vi "Configure Zone.vi"(0 "VISA resource name":refnum<visa-resource-name>, 1 "Manual\nOutput (0.000)":dbl[](array[numeric]) min=-100.0 max=100.0 step=0.001 format="%.3f", 2 "Heater\nRange (0: Off)":i8[](array[ring]) items=["Off", "Low (0.5W)", "Med (5W)", "High (50W)"], 5 "Loop (0: 1)":u16(ring) items=["1", "2"], 9 "Top \nValue (0.0000)":dbl[](array[numeric]) min=-273.0 max=1500.0 step=0.0001 format="%.4f", 11 "error in (no error)":errorcluster, 12 "Gain (0.0)":dbl[](array[numeric]) min=0.0 max=1000.0 step=0.1 format="%.1f", 13 "Reset (0.0)":dbl[](array[numeric]) min=0.0 max=1000.0 step=0.1 format="%.1f", 14 "Rate (0)":dbl[](array[numeric]) min=0.0 max=200.0 step=1.0) -> (4 "VISA resource name out":refnum<visa-resource-name>, 6 "Zone":i32[](array[numeric]) min=1 max=10 step=1, 15 "error out":errorcluster)   [LabVIEW 2013, in "Lake Shore Cryotronics 331.lvlib"]
doc: "This VI Configures the parameters of a control loop's zone table. The zone values are configured into arrays to allow all ten zones to be sent each time the vi is executed."
uses:
  Lake Shore Cryotronics 331.lvlib
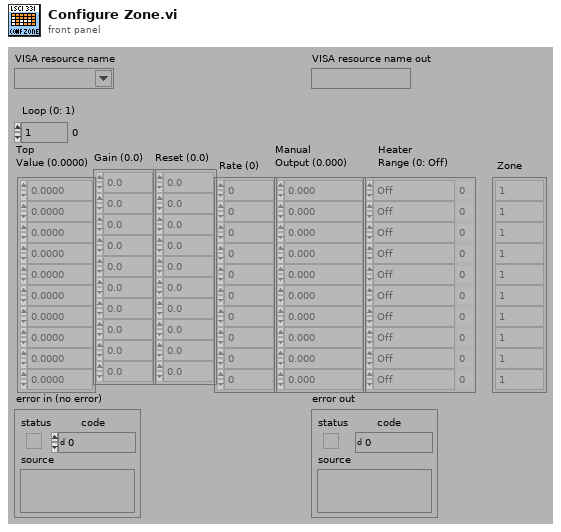
[diagram p1: front panel]
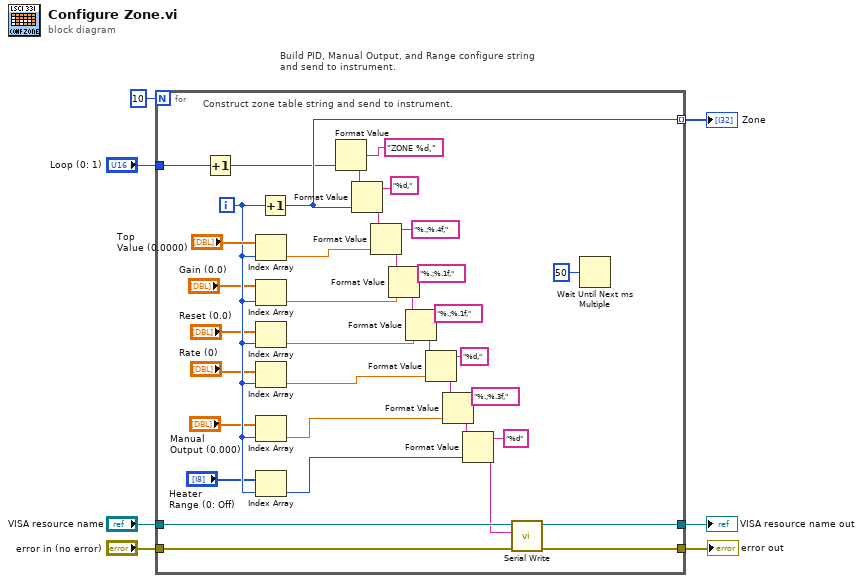
[diagram p0: block diagram]
diagram:
  # "Build PID, Manual Output, and Range configure string\nand send to instrument."
  n1 = for {
    N: 10 -> [_]
    tunnel: [w28] -> w6 mode=indexing
    tunnel: "Loop (0: 1)" -> [w25]
    tunnel: "error in (no error)" -> [w13]
    tunnel: [w12] -> w4
    tunnel: [w11] -> w3
    tunnel: "VISA resource name" -> [w9]
    i -> [w22]
    # "Construct zone table string and send to instrument."
    n2 = Increment(x=w25) -> (x+1=w10:u16)
    n3 = Index Array(array="Top \nValue (0.0000)", index=w22) -> (element=w33:dbl)
    n4 = Index Array(array="Gain (0.0)", index=w22) -> (element=w32:dbl)
    n5 = Index Array(array="Reset (0.0)", index=w22) -> (element=w31:dbl)
    n6 = Index Array(array="Rate (0)", index=w22) -> (element=w30:dbl)
    n7 = Index Array(array="Manual\nOutput (0.000)", index=w22) -> (element=w29:dbl)
    n8 = Index Array(array="Heater\nRange (0: Off)", index=w22) -> (element=w18:i8)
    n9 = Increment(x=w22) -> (x+1=w28:i32)
    n10 = Format Value(format string="ZONE %d,", value (0)=w10) -> (output string=w24:string)  [unwired: 1 in]
    n11 = Format Value(string ("")=w24, format string="%d,", value (0)=w28) -> (output string=w35:string)
    n12 = Format Value(string ("")=w35, format string="%.;%.4f,", value (0)=w33) -> (output string=w41:string)
    n13 = Format Value(string ("")=w41, format string="%.;%.1f,", value (0)=w32) -> (output string=w42:string)
    n14 = Format Value(string ("")=w42, format string="%.;%.1f,", value (0)=w31) -> (output string=w43:string)
    n15 = Format Value(string ("")=w43, format string="%d,", value (0)=w30) -> (output string=w44:string)
    n16 = Format Value(string ("")=w44, format string="%.;%.3f,", value (0)=w29) -> (output string=w19:string)
    n17 = Format Value(string ("")=w19, format string="%d", value (0)=w18) -> (output string=w8:string)
    n18 = call "Serial Write.vi"("error in (no error)"=w13, "Write Buffer (\"\")"=w8, "VISA resource name"=w9) -> ("error out"=w11:errorcluster, "VISA resource name out"=w12:refnum<visa-resource-name>)  [unwired: 6 in, 1 out]
    n19 = Wait Until Next ms Multiple(millisecond multiple=u32 50) -> ()  [unwired: 1 out]
  }
  "Zone" <- w6
  "VISA resource name out" <- w4
  "error out" <- w3
